vi "ln.vi"(8 "ready for output (T)":bool=TRUE, 9 "input valid":bool, 10 "x":fxp<+/-,64,32>) -> (0 "ready for input":bool, 1 "output valid":bool, 2 "ln(x)":fxp<+/-,32,16>)   [LabVIEW 2018]
uses:
  <vilib>/rvi/FXPMathLib/FxpLn/subVIs/nifxpmath_NaturalLogarithm_SimConfig.ctl
  <vilib>/rvi/FXPMathLib/FxpLn/simVIs/DllFxpNaturalLogarithmTemp_sub.vi
  <vilib>/rvi/FXPMathLib/FxpMul/XNode/nifxpmath_Multiplier.xnode
  <vilib>/rvi/FXPMathLib/FxpLn/XNode/nifxpmath_NaturalLogarithm.xnode
  <vilib>/rvi/FXPMathLib/FxpAdd/XNode/nifxpmath_Add.xnode
  <vilib>/rvi/FXPMathLib/sim/FxpSim.dll
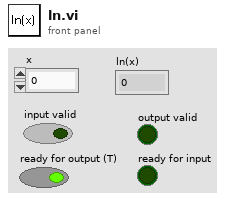
[diagram p1: front panel]
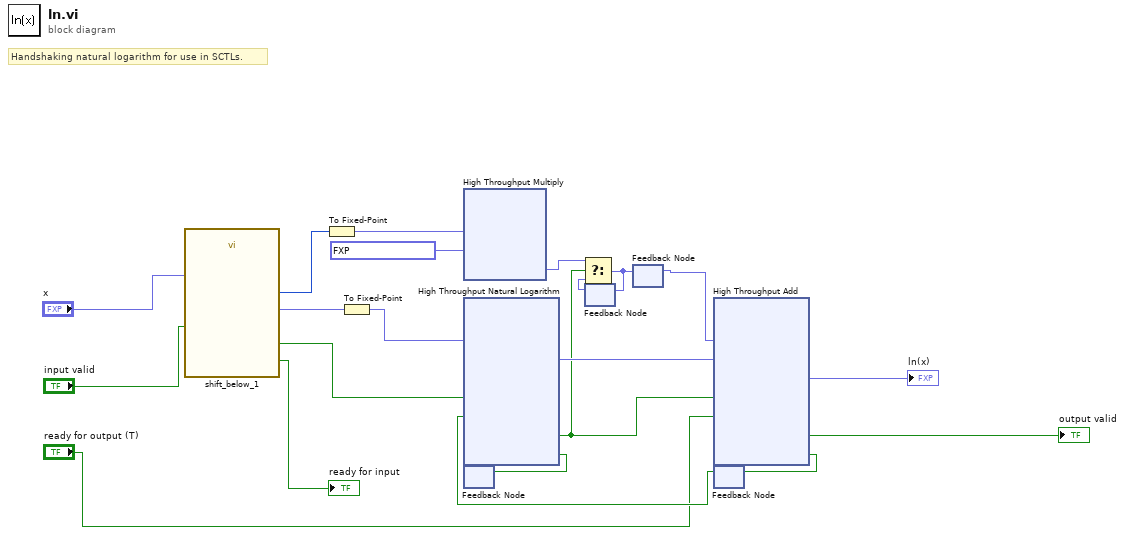
[diagram p0: block diagram]
diagram:
  # "Handshaking natural logarithm for use in SCTLs."
  n1 = call "shift_below_1.vi"("input valid"="input valid", "input"="x") -> ("ready for input"=→"ready for input":bool, "output valid"=w3:bool, "shifted"=w20:fxp<+/-,64,32>, "count"=w14:i16)  [unwired: 6 in]
  n2 = To Fixed-Point(number=w14) -> (fixed-point=w12:fxp<+,8,8>)  [unwired: 1 in]
  n3 = To Fixed-Point(number=w20) -> (fixed-point=w19:fxp<+,16,0>)  [unwired: 1 in]
  n4 = xnode "High Throughput Multiply"("x"=w12, "y"=fxp<+,32,16> 0.693145751953125) -> ("x*y"=w8:fxp<+,40,24>)
  n5 = feedback #1() -> ()  [unwired: 2 in]
  n6 = feedback #2() -> (w7:fxp<+,40,24>)  [unwired: 1 in]
  n7 = feedback #3() -> (w5:fxp<+,40,24>)  [unwired: 1 in]
  n8 = feedback #4() -> (w11:bool)  [unwired: 1 in]
  n9 = xnode "High Throughput Natural Logarithm"("x"=w19, "input valid"=w3, "ready for output (T)"=w11) -> ("ln(x)"=w15:fxp<+/-,16,1>, "output valid"=w1:bool, "ready for input"=w9:bool)  [unwired: 1 out]
  n10 = feedback-in #1(w9) -> ()
  n11 = Select(t=w8, s=w1, f=w7) -> (s? t:f=w6:fxp<+,40,24>)
  n12 = feedback-in #2(w6) -> ()
  n13 = feedback-in #3(w6) -> ()
  n14 = xnode "High Throughput Add"("x"=w5, "y"=w15, "input valid"=w1, "ready for output (T)"="ready for output (T)") -> ("x+y"=→"ln(x)":fxp<+/-,42,26>, "output valid"=→"output valid":bool, "ready for input"=w16:bool)
  n15 = feedback-in #4(w16) -> ()
